vi "WebVGA click demo.vi"(10 "Column":u8, 11 "Row":u8) -> ()   [LabVIEW 2014]
uses:
  Global vars.vi
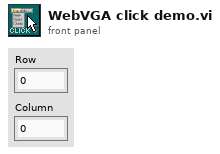
[diagram p1: front panel]
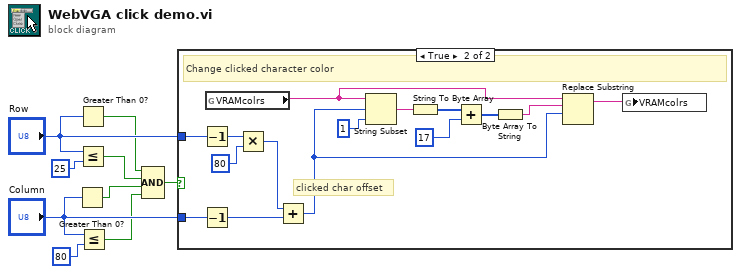
[diagram p0: block diagram]
diagram:
  n1 = Greater Than 0?(x="Column") -> (x > 0?=w3:bool)
  n2 = Greater Than 0?(x="Row") -> (x > 0?=w5:bool)
  n3 = Less Or Equal?(x="Row", y=u8 25) -> (x <= y?=w4:bool)
  n4 = Less Or Equal?(x="Column", y=u8 80) -> (x <= y?=w2:bool)
  n5 = Compound Arithmetic op=AND(w5, w4, w3, w2) -> (w1:bool)
  n6 = case shown="True" w1 {
    tunnel: "Column" -> [_ w20]
    tunnel: "Row" -> [_ w19]
    frame False {
    }
    frame True {
      # "clicked char offset"
      # "Change clicked character color"
      n7 = Decrement(x=w19) -> (x-1=w24:u8)
      n8 = Decrement(x=w20) -> (x-1=w21:u8)
      n9 = global read "Global vars.vi" "VRAMcolrs"() -> (w13:string)
      n10 = Multiply(x=w24, y=80) -> (x*y=w22:i32)
      n11 = Add(x=w22, y=w21) -> (x+y=w11:i32)
      n12 = String Subset(string=w13, offset (0)=w11, length (rest)=1 ("length (rest)")) -> (substring=w17:string)
      n13 = String To Byte Array(string=w17) -> (unsigned byte array=w15:u8[])
      n14 = Add(x=w15, y=u8 17) -> (x+y=w14:u8[])
      n15 = Byte Array To String(unsigned byte array=w14) -> (string=w12:string)
      n16 = Replace Substring(3:w11, 4:w12, 5:w13) -> (1:w10:string)  [unwired: 1 in, 1 out]
      n17 = global write "Global vars.vi" "VRAMcolrs"(w10) -> ()
    }
  }
